vi "1.vi"() -> ()   [LabVIEW 2016]
panel:
  out "x/y":dbl
  out "x*y":dbl
  out "x-y":dbl
  out "x+y":dbl
  out "Boolean":bool
  in  "y":dbl
  in  "x":dbl
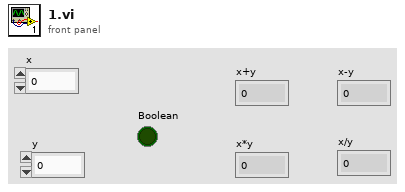
[diagram p1: front panel]
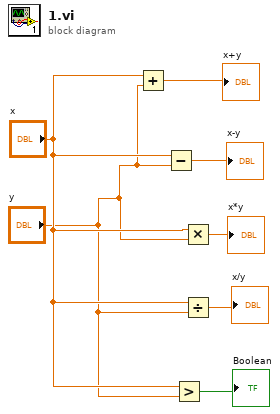
[diagram p0: block diagram]
diagram:
  n1 = Add(x="x", y="y") -> (x+y=→"x+y":dbl)
  n2 = Subtract(x="x", y="y") -> (x-y=→"x-y":dbl)
  n3 = Greater?(x="x", y="y") -> (0:→"Boolean":bool)
  n4 = Multiply(x="x", y="y") -> (x*y=→"x*y":dbl)
  n5 = Divide(x="x", y="y") -> (x/y=→"x/y":dbl)
